vi "processData.vi"(3 "Cursor List":T1, 4 "data in":dbl[][][](array[numeric])) -> (0 "Angle Chart":dbl[][](array[numeric]), 1 "Energy Chart":dbl[][](array[numeric]), 2 "Intensity Chart":dbl[](array[numeric]))   [LabVIEW 2020]
uses:
  <vilib>/Utility/miscctls.llb/LVCursorListTypeDef.ctl
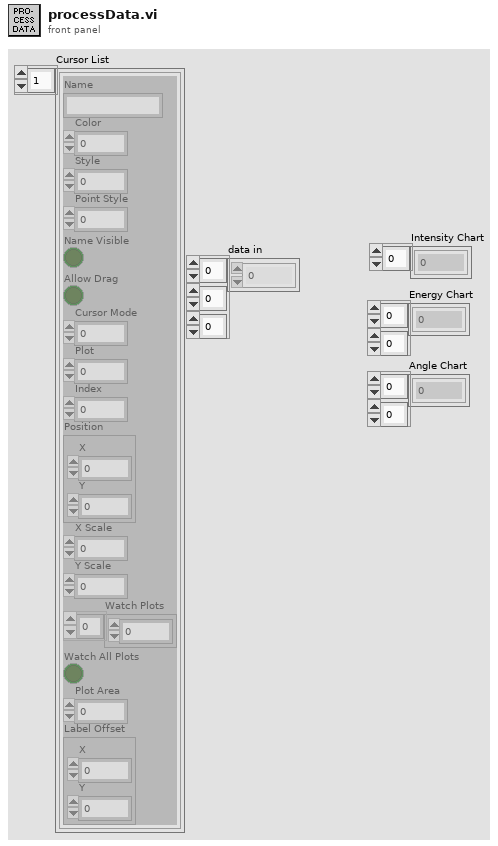
[diagram p1: front panel]
types:
  T1 = typedef "LVCursorListTypeDef.ctl" = cluster{"Name":string, "Color":u32, "Style":u8, "Point Style":u8, "Name Visible":bool, "Allow Drag":bool, "Cursor Mode":u32, "Plot":i32, "Index":i32, "Position":cluster{"X":dbl, "Y":dbl}, "X Scale":u32, "Y Scale":u32, "Watch Plots":i32[], "Watch All Plots":bool, "Plot Area":i32, "Label Offset":cluster{"X":dbl, "Y":dbl}}[]
  T2 = cluster{"Name":string, "Color":u32, "Style":u8, "Point Style":u8, "Name Visible":bool, "Allow Drag":bool, "Cursor Mode":u32, "Plot":i32, "Index":i32, "Position":cluster{"X":dbl, "Y":dbl}, "X Scale":u32, "Y Scale":u32, "Watch Plots":i32[], "Watch All Plots":bool, "Plot Area":i32, "Label Offset":cluster{"X":dbl, "Y":dbl}}
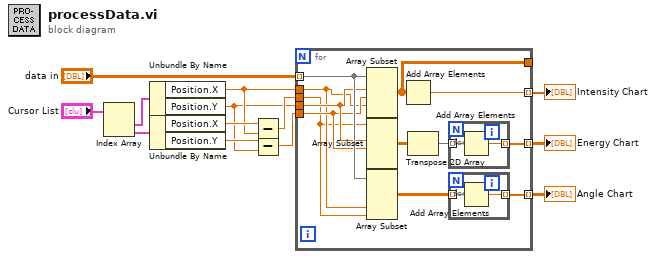
[diagram p0: block diagram]
diagram:
  n1 = Index Array(array="Cursor List") -> (element #1=w12:T2, element #2=w13:T2)  [unwired: 2 in]
  n2 = Unbundle By Name(w12) -> ("Position.X"=w7:dbl, "Position.Y"=w5:dbl)
  n3 = Unbundle By Name(w13) -> ("Position.X"=w10:dbl, "Position.Y"=w9:dbl)
  n4 = Subtract(x=w10, y=w7) -> (x-y=w6:dbl)
  n5 = Subtract(x=w9, y=w5) -> (x-y=w4:dbl)
  n6 = for {
    tunnel: "data in" -> [w19] mode=indexing
    tunnel: w7 -> [w15]
    tunnel: w6 -> [w14]
    tunnel: [w25] -> w3 mode=indexing
    tunnel: w5 -> [w17]
    tunnel: w4 -> [w16]
    tunnel: [w21] -> w2 mode=indexing
    tunnel: [w20] -> w1 mode=indexing
    tunnel: [w18] -> _
    n7 = Array Subset(array=w19, index (row)=w17, length (row)=w16, index (col)=w15, length (col)=w14) -> (w18:dbl[][])
    n8 = Array Subset(array=w19, index (row)=w17, length (row)=w16) -> (w24:dbl[][])  [unwired: 2 in]
    n9 = Array Subset(array=w19, index (col)=w15, length (col)=w14) -> (w22:dbl[][])  [unwired: 2 in]
    n10 = Add Array Elements(numeric array=w18) -> (sum=w25:dbl)
    n11 = Transpose 2D Array(2D array=w24) -> (transposed array=w23:dbl[][])
    n12 = for {
      tunnel: w23 -> [w28] mode=indexing
      tunnel: [w29] -> w21 mode=indexing
      n13 = Add Array Elements(numeric array=w28) -> (sum=w29:dbl)
    }
    n14 = for {
      tunnel: w22 -> [w26] mode=indexing
      tunnel: [w27] -> w20 mode=indexing
      n15 = Add Array Elements(numeric array=w26) -> (sum=w27:dbl)
    }
  }
  "Energy Chart" <- w2
  "Angle Chart" <- w1
  "Intensity Chart" <- w3
